vi "Disabled.vi"(8 "error in (no error)":errorcluster, 11 "Elevator Concrete in":refnum<class "Elevator Arm.lvclass">) -> (0 "error out":errorcluster, 3 "Elevator Concrete out":refnum<class "Elevator Arm.lvclass">)   [LabVIEW 2019, in "Elevator.lvlib" / "Elevator Arm.lvclass"]
doc: "Disable Motors\nThis method sets the elevator arm motors to percent output mode with 0 output.\nThis prevents motion magic drive from retaining P and going immediately to\n100% percent when re-enabled."
uses:
  Elevator Arm.lvclass
  <vilib>/Rock Robotics/WPI/ThirdParty/Phoenix-LabVIEW/Motor Controller/Controls/CTRE_Phoenix_MotorControl_ControlMode.ctl
  Elevator Arm.lvclass/Elevator Arm.ctl
  Elevator.lvclass
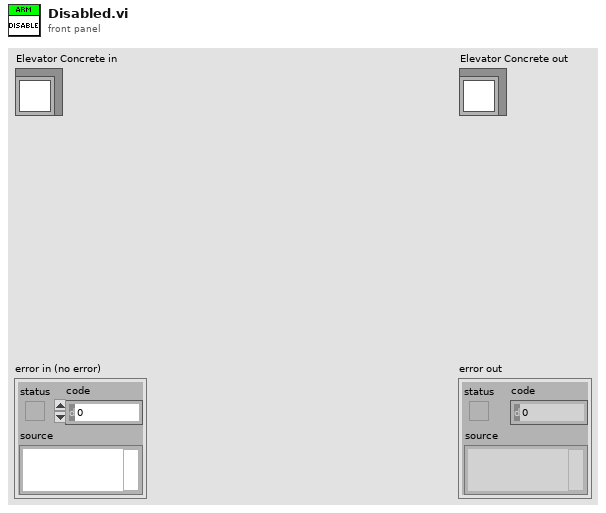
[diagram p1: front panel]
types:
  T1 = typedef "CTRE_Phoenix_MotorControl_ControlMode.ctl" = u16
  T2 = typedef "WPI_MotorControlDeviceRef.ctl" = cluster{"DeviceStatus":errorcluster, "Type":T3, "PWM":cluster{"PWM Channel":T4, "DeadBand":T5}, "CAN":cluster{"Device Number":u8, "SetOutput VI Ref":variant, "GetOutput VI Ref":variant, "Enable VI Ref":variant, "Disable VI Ref":variant, "Data":variant}, "Invert":bool, "DIO PWM":cluster{"PWM \"Enable\" Channel":T4, "DIOChannel":T6, "PWM Rate":dbl}}
  T3 = typedef "WPI_MotorControlType.ctl" = enum16{"PWM", "CAN", "DIO PWM"}
  T4 = typedef "FPGA_DIOPWMChannel.ctl" = enum8{"PWM 0", "PWM 1", "PWM 2", "PWM 3", "PWM 4", "PWM 5", "PWM 6", "PWM 7", "PWM 8", "PWM 9", "PWM MXP 0", "PWM MXP 1", "PWM MXP 2", "PWM MXP 3", "PWM MXP 4", "PWM MXP 5", "PWM MXP 6", "PWM MXP 7", "PWM MXP 8", "PWM MXP 9", "Invalid"}
  T5 = typedef "WPI_PWMDeadband.ctl" = cluster{"Name":string, "maxPositivePwm":i32, "minPositivePwm":i32, "centerPwm":i32, "maxNegativePwm":i32, "minNegativePwm":i32, "angularRange":u16}
  T6 = typedef "FPGA_DIOChannel.ctl" = enum8{"DIO 0", "DIO 1", "DIO 2", "DIO 3", "DIO 4", "DIO 5", "DIO 6", "DIO 7", "DIO 8", "DIO 9", "DIO MXP 0", "DIO MXP 1", "DIO MXP 2", "DIO MXP 3", "DIO MXP 4", "DIO MXP 5", "DIO MXP 6", "DIO MXP 7", "DIO MXP 8", "DIO MXP 9", "DIO MXP 10", "DIO MXP 11", "DIO MXP 12", "DIO MXP 13", "DIO MXP 14", "DIO MXP 15", "SPI Port CS1", "SPI Port CS2", "SPI Port CS3", "SPI Port MISO", "SPI Port MOSI", "Invalid"}
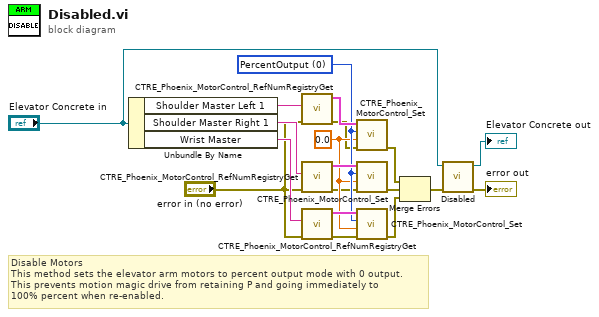
[diagram p0: block diagram]
diagram:
  w11 = 0.0 ("Output")
  w12 = T1 0 items=["PercentOutput"=0, "Position"=1, "Velocity"=2, "Current"=3, "Follower"=5, "MotionProfile"=6, "MotionMagic"=7, "MotionProfileArc"=10, "Disabled"=15] ("Control Mode")
  # "Disable Motors\nThis method sets the elevator arm motors to percent output mode with 0 output.\nThis prevents motion magic drive from retaining P and going immediately to\n100% percent when re-enabled."
  n1 = Unbundle By Name("Elevator Concrete in") -> ("Shoulder Master Left 1"=w7:string, "Shoulder Master Right 1"=w15:string, "Wrist Master"=w6:string)
  n2 = call <vilib>:"CTRE_Phoenix_MotorControl_RefNumRegistryGet.vi"("error in (no error)"="error in (no error)", "refnum name"=w7) -> ("error out"=w10:errorcluster, "PhoenixMotorControlDevRef"=w16:T2)  [unwired: 8 in]
  n3 = call <vilib>:"CTRE_Phoenix_MotorControl_RefNumRegistryGet.vi"("error in (no error)"="error in (no error)", "refnum name"=w15) -> ("error out"=w9:errorcluster, "PhoenixMotorControlDevRef"=w14:T2)  [unwired: 8 in]
  n4 = call <vilib>:"CTRE_Phoenix_MotorControl_RefNumRegistryGet.vi"("error in (no error)"="error in (no error)", "refnum name"=w6) -> ("error out"=w8:errorcluster, "PhoenixMotorControlDevRef"=w13:T2)  [unwired: 8 in]
  n5 = call <vilib>:"CTRE_Phoenix_MotorControl_Set.vi"("error in (no error)"=w10, "Output"=w11, "Control Mode"=w12, "PhoenixMotorControlDevRef"=w16) -> ("error out"=w4:errorcluster)  [unwired: 6 in, 1 out]
  n6 = call <vilib>:"CTRE_Phoenix_MotorControl_Set.vi"("error in (no error)"=w9, "Output"=w11, "Control Mode"=w12, "PhoenixMotorControlDevRef"=w14) -> ("error out"=w3:errorcluster)  [unwired: 6 in, 1 out]
  n7 = call <vilib>:"CTRE_Phoenix_MotorControl_Set.vi"("error in (no error)"=w8, "Output"=w11, "Control Mode"=w12, "PhoenixMotorControlDevRef"=w13) -> ("error out"=w2:errorcluster)  [unwired: 6 in, 1 out]
  n8 = Merge Errors(w4, w3, w2) -> (w1:errorcluster)
  n9 = call-parent "Disabled.vi"("error in (no error)"=w1, "Elevator in"="Elevator Concrete in") -> ("error out"=→"error out":errorcluster, "Elevator out"=→"Elevator Concrete out":refnum<class "Elevator Arm.lvclass">)  [unwired: 8 in]
